vi "Compass on new GIC B.vi"(11 "GIC Input":T1={"     Use ?\nOff       On"=[FALSE, TRUE, FALSE, TRUE], "Mode:"=FALSE, "Extra Port"="", "Hokuyo Port"="COM7", "Tx Prop  Port"="COM6", "Compass Port"="", "GPS Port"="", "Num of WPs"=0, "WP Lats and Longs"={"WP Lats"=[], "WP Longs"=[]}, "Obst Lats and Longs"={"Obst Lats"=[], "Obst Longs"=[]}, "Parameters"=[], "GPS Data"=[], "Compass"=0.0, "LMS Vector"=[], "Vision Vector"=[], "Direction Cmd"=0.0, "Speed Cmd"=0.0, "WP Vector"=[], "WP Number"=0, "Extra"=0, "SW Map"=[], "Path Cluster"={"Path x node"=[], "Path y node"=[]}, "Sim Course"=[]} {"Obst Lats and Longs"."Obst Longs" format="%#_8g"; "Obst Lats and Longs"."Obst Lats" format="%#_8g"}) -> (3 "GIC Output":T1={"     Use ?\nOff       On"=[FALSE, TRUE, FALSE, TRUE], "Mode:"=FALSE, "Extra Port"="", "Hokuyo Port"="COM7", "Tx Prop  Port"="COM6", "Compass Port"="", "GPS Port"="", "Num of WPs"=0, "WP Lats and Longs"={"WP Lats"=[], "WP Longs"=[]}, "Obst Lats and Longs"={"Obst Lats"=[], "Obst Longs"=[]}, "Parameters"=[], "GPS Data"=[], "Compass"=0.0, "LMS Vector"=[], "Vision Vector"=[], "Direction Cmd"=0.0, "Speed Cmd"=0.0, "WP Vector"=[], "WP Number"=0, "Extra"=0, "SW Map"=[], "Path Cluster"={"Path x node"=[], "Path y node"=[]}, "Sim Course"=[]} {"Obst Lats and Longs"."Obst Longs" format="%#_8g"; "Obst Lats and Longs"."Obst Lats" format="%#_8g"})   [LabVIEW 2014]
panel:
  out "compass out":dbl
  # "Compass on New GIC B"
  # "Input:"
  # "Output:"
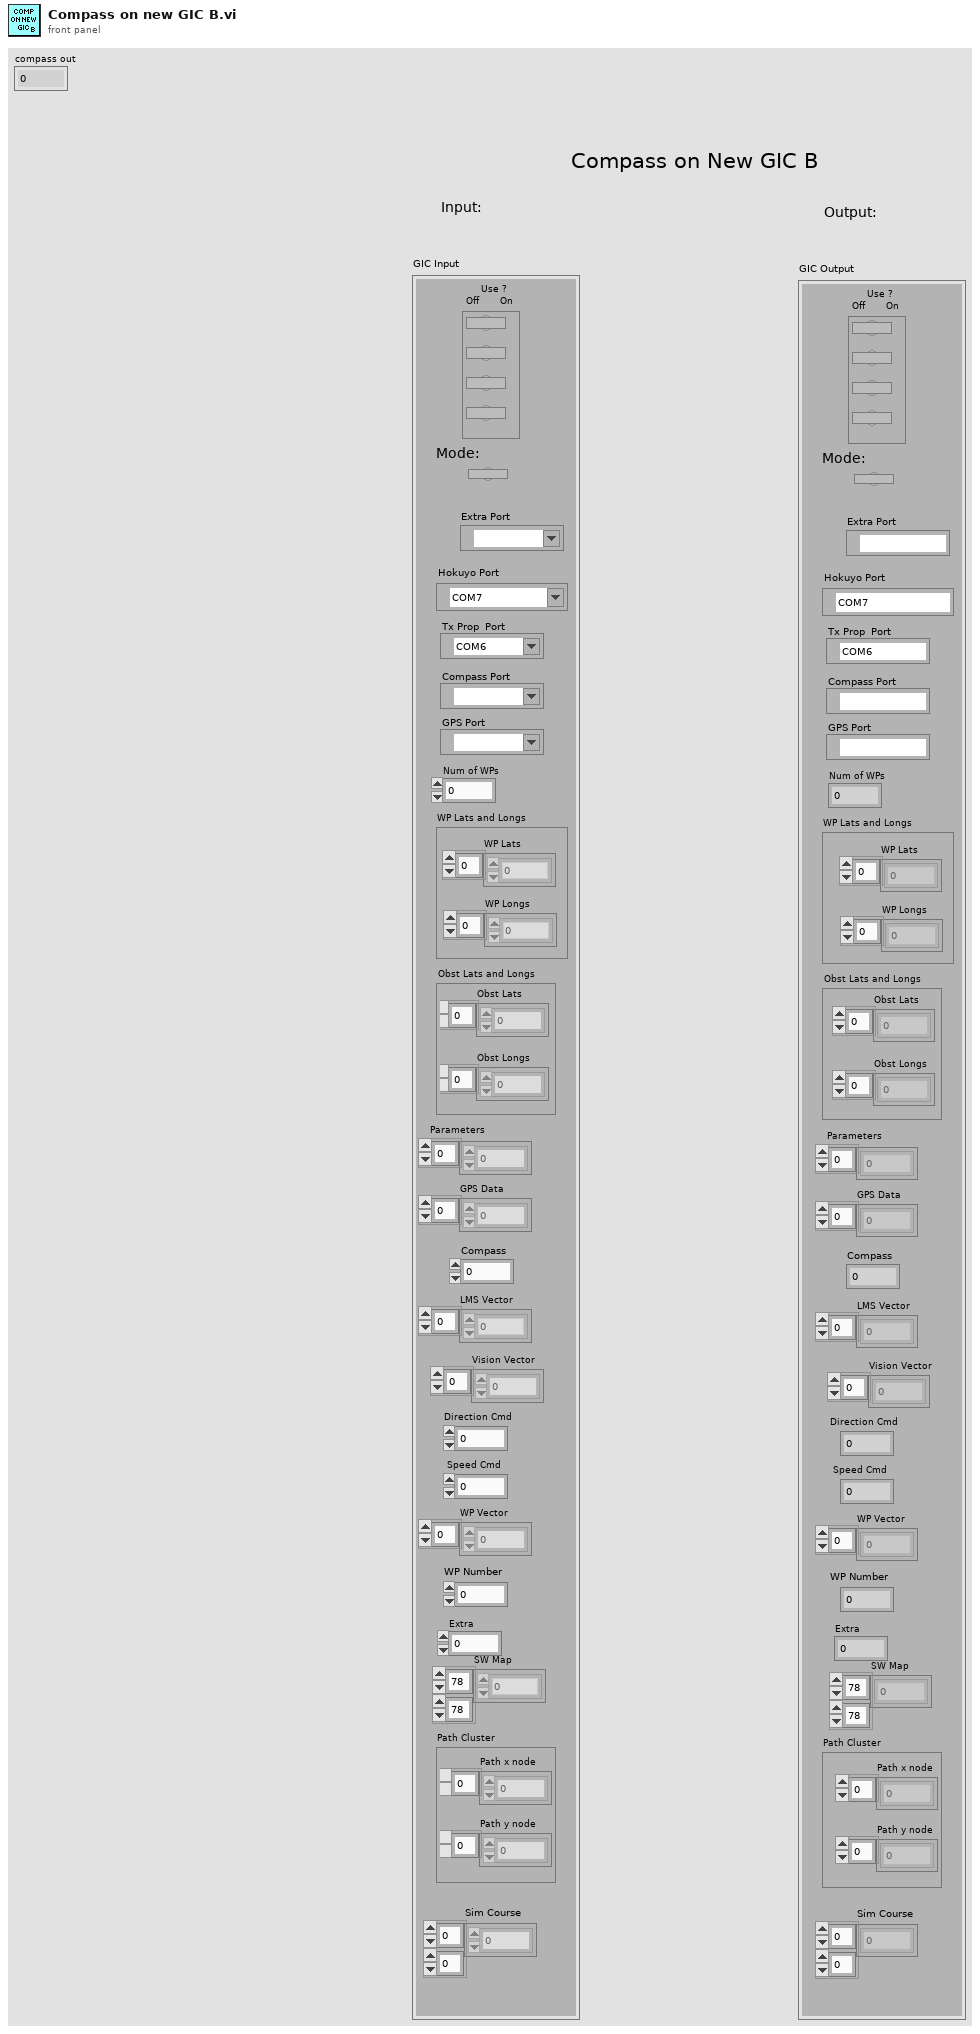
[diagram p1: front panel]
types:
  T1 = cluster{"     Use ?\nOff       On":bool[], "Mode:":bool, "Extra Port":refnum<visa-resource-name>, "Hokuyo Port":refnum<visa-resource-name>, "Tx Prop  Port":refnum<visa-resource-name>, "Compass Port":refnum<visa-resource-name>, "GPS Port":refnum<visa-resource-name>, "Num of WPs":i16, "WP Lats and Longs":cluster{"WP Lats":dbl[], "WP Longs":dbl[]}, "Obst Lats and Longs":cluster{"Obst Lats":dbl[], "Obst Longs":dbl[]}, "Parameters":dbl[], "GPS Data":dbl[], "Compass":dbl, "LMS Vector":dbl[], "Vision Vector":dbl[], "Direction Cmd":dbl, "Speed Cmd":dbl, "WP Vector":dbl[], "WP Number":i32, "Extra":i16, "SW Map":i32[][], "Path Cluster":cluster{"Path x node":dbl[], "Path y node":dbl[]}, "Sim Course":i8[][]}
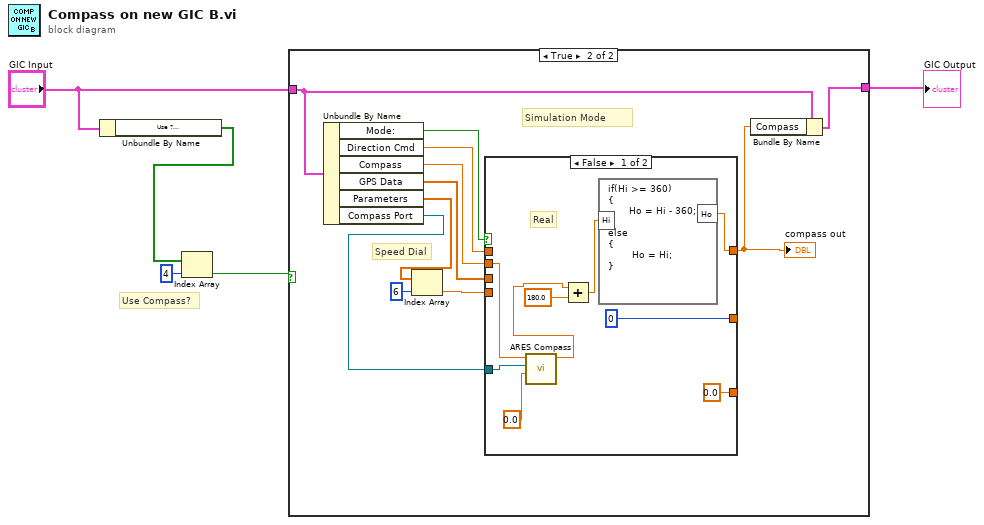
[diagram p0: block diagram]
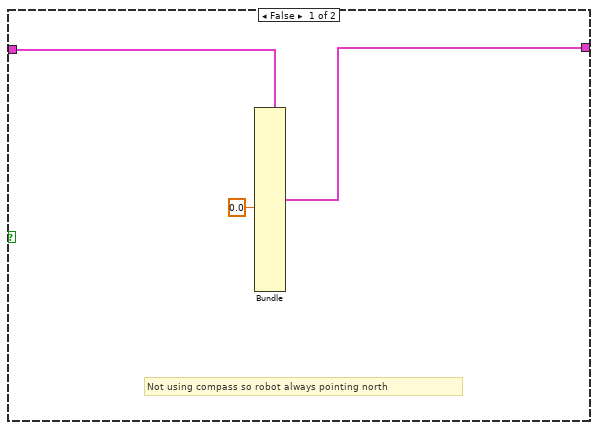
[diagram p2: hidden frame]
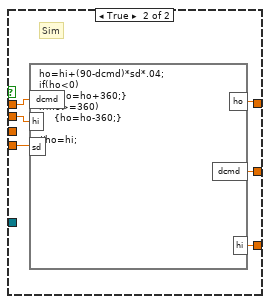
[diagram p3: hidden frame]
diagram:
  # "Use Compass?"
  n1 = Unbundle By Name("GIC Input") -> ("Use ?\nOff       On"=w5:bool[])
  n2 = Index Array(array=w5, index=4) -> (element=w3:bool)
  n3 = case shown="True" w3 {
    tunnel: "GIC Input" -> [w8 w14]
    tunnel: [w6 w13] -> w1
    frame False {
      # "Not using compass so robot always pointing north"
      n4 = Bundle(cluster=w8, "Compass"=0.0) -> (w6:T1)  [unwired: 22 in]
    }
    frame True {
      # "Simulation Mode"
      # "Speed Dial"
      n5 = Unbundle By Name(w14) -> ("Mode:"=w18:bool, "Direction Cmd"=w12:dbl, "Compass"=w11:dbl, "GPS Data"=w19:dbl[], "Parameters"=w17:dbl[], "Compass Port"=w9:refnum<visa-resource-name>)
      n6 = Index Array(array=w17, index=6) -> (element=w15:dbl)
      n7 = case shown="False" w18 {
        tunnel: w12 -> [_ w33]
        tunnel: w11 -> [w26 w32]
        tunnel: [w21 w34] -> w10
        tunnel: w19 -> [_ _]
        tunnel: w15 -> [_ w31]
        tunnel: [0 w30] -> _
        tunnel: [0.0 ("hi") w29] -> _
        tunnel: w9 -> [w25 _]
        frame False {
          # "Real"
          n8 = call "ARES Compass.vi"("Input time of last compass read"=0.0, "Compass Com Port"=w25, "Compass In"=w26) -> ("Compass Out"=w22:dbl)  [unwired: 6 in, 1 out]
          n9 = Add(x=w22, y=180.0) -> (x+y=w20:dbl)
          n10 = formula code="if(Hi >= 360)\n{\n       Ho = Hi - 360;\n}\nelse\n{\n        Ho = Hi;\n}"("Hi"=w20) -> ("Ho"=w21:dbl)
        }
        frame True {
          # "Sim"
          n11 = formula code="ho=hi+(90-dcmd)*sd*.04;\nif(ho<0)\n     {ho=ho+360;}\nif(ho>=360)\n     {ho=ho-360;}\n\n//ho=hi;"("dcmd"=w33, "hi"=w32, "sd"=w31) -> ("ho"=w34:dbl, "dcmd"=w30:dbl, "hi"=w29:dbl)
        }
      }
      "compass out" <- w10
      n12 = Bundle By Name(cluster=w14, "Compass"=w10) -> (w13:T1)
    }
  }
  "GIC Output" <- w1
